vi "Start.vi"(8 "error in (no error)":errorcluster) -> (0 "error out":errorcluster)   [LabVIEW 2018, in "GLog.lvlib" / "Registry.lvlib"]
uses:
  Registry.lvlib
  Registry Message.ctl
  Registry Actions.ctl
  Registry Actions Event.vi
  Registry.vi
  <vilib>/Utility/error.llb/Error Cluster From Error Code.vi
  <vilib>/ErrorRing/Error Ring.xnode
  reuse_library/Utilities/Utilities.lvlib
panel:
  # "Connector Pane"
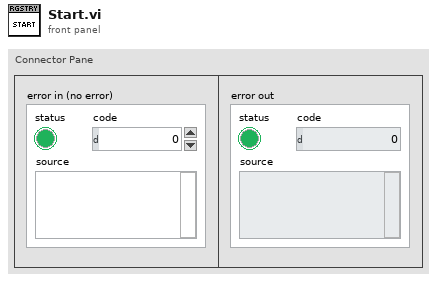
[diagram p1: front panel]
types:
  T1 = typedef "GLog.lvlib/Registry.lvlib/Registry Message.ctl" = cluster{"action":T2, "data":variant, "return notifier":refnum<notifier>}
  T2 = typedef "GLog.lvlib/Registry.lvlib/Registry Actions.ctl" = enum16{"Register", "Log", "Enable", "Enable All", "Disable", "Disable All", "List", "Unregister", "Unregister All", "Shutdown"}
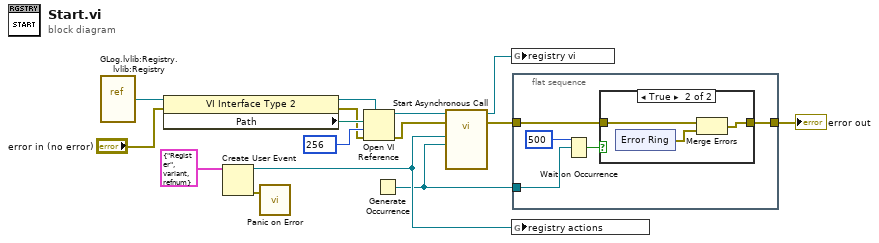
[diagram p0: block diagram]
diagram:
  n1 = vi-ref "GLog.lvlib:Registry.lvlib:Registry.vi"() -> (w13:refnum<vi>)
  n2 = property class="VI Interface Type 2"(reference=w13, error in="error in (no error)") -> (reference out=w12:refnum<vi>, error out=w6:errorcluster, "Path"=w14:path)
  n3 = Create User Event(user event datatype=T1 {"action"=enum."Register", "data"=variant, "return notifier"=refnum} ("registry message")) -> (user event=w10:refnum<user-event>, error out=w9:errorcluster)  [unwired: 1 in]
  n4 = call "Panic on Error.vi"("error in (no error)"=w9) -> ()  [unwired: 3 in]
  n5 = Open VI Reference(type specifier VI Refnum (for type only)=w12, vi path=w14, options=256, error in (no error)=w6) -> (vi reference=w5:refnum<vi>, error out=w7:errorcluster)  [unwired: 2 in]
  n6 = Generate Occurrence() -> (w2:refnum<k4>)
  n7 = call-by-ref "Start Asynchronous Call"(reference=w5, error in=w7, "setup occurrence"=w2, "registry actions"=w10) -> (reference out=w1:refnum<vi>, error out=w3:errorcluster)  [unwired: 10 in]
  n8 = global write "Registry Actions Event.vi" "registry vi"(w1) -> ()
  n9 = global write "Registry Actions Event.vi" "registry actions"(w10) -> ()
  n10 = flat-sequence {
    tunnel: w2 -> [w20]
    tunnel: [w17] -> w4
    tunnel: w3 -> [w16]
    frame #0 {
      n11 = Wait on Occurrence(2:w20, 3:500 ("ms timeout (-1)")) -> (0:w18:bool)  [unwired: 1 in]
      n12 = case shown="True" w18 {
        tunnel: [w21 w23] -> w17
        tunnel: w16 -> [w21 w24]
        frame False {
        }
        frame True {
          n13 = xnode "Error Ring"() -> ("error out"=w22:errorcluster)
          n14 = Merge Errors(w24, w22) -> (w23:errorcluster)
        }
      }
    }
  }
  "error out" <- w4
